vi "SR_FlipFlop_Example.vi"() -> ()   [LabVIEW 2019]
uses:
  <vilib>/Rock Robotics/WPI/ThirdParty/JAS_Junk/TrajLib/Trajectory_Library.lvlib
panel:
  in  "Set":bool
  in  "Reset":bool
  out "Output":bool
  out "NOT Output":bool
  out "Digital State Chart":cluster{dbl, dbl, dbl, dbl}(graph)
  # "S/R (Set/Reset) Flip-Flop Example"
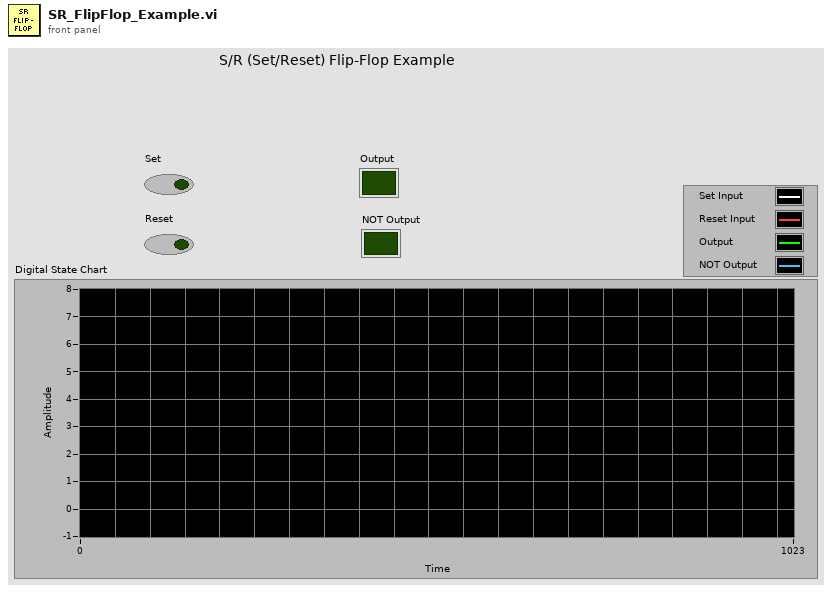
[diagram p1: front panel]
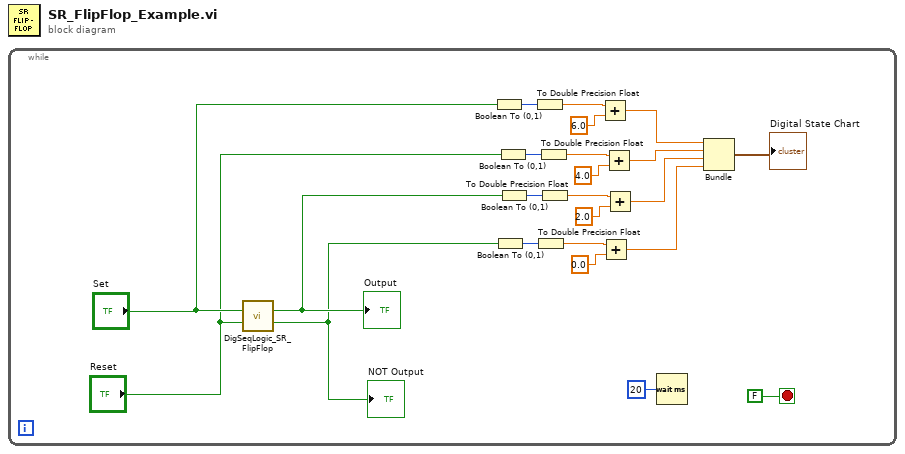
[diagram p0: block diagram]
diagram:
  n1 = while {
    stop <- FALSE stop-if-true
    n2 = call <vilib>:"DigSeqLogic_SR_FlipFlop.vi"("Set"="Set", "Reset"="Reset") -> ("Output"=w5:bool, "Inverse Output"=w4:bool)  [unwired: 12 in]
    "Output" <- w5
    "NOT Output" <- w4
    n3 = Boolean To (0,1)(Boolean="Set") -> (0, 1=w10:i16)
    n4 = Boolean To (0,1)(Boolean=w4) -> (0, 1=w11:i16)
    n5 = Boolean To (0,1)(Boolean="Reset") -> (0, 1=w13:i16)
    n6 = Boolean To (0,1)(Boolean=w5) -> (0, 1=w15:i16)
    n7 = To Double Precision Float(number=w10) -> (double precision float=w20:dbl)
    n8 = To Double Precision Float(number=w11) -> (double precision float=w12:dbl)
    n9 = To Double Precision Float(number=w13) -> (double precision float=w14:dbl)
    n10 = To Double Precision Float(number=w15) -> (double precision float=w16:dbl)
    n11 = Add(x=w20, y=6.0) -> (x+y=w21:dbl)
    n12 = Add(x=w12, y=0.0) -> (x+y=w19:dbl)
    n13 = Add(x=w14, y=4.0) -> (x+y=w17:dbl)
    n14 = Add(x=w16, y=2.0) -> (x+y=w18:dbl)
    n15 = Wait (ms)(milliseconds to wait=u32 20) -> ()  [unwired: 1 out]
    n16 = Bundle(w21, w17, w18, w19) -> (→"Digital State Chart":cluster{dbl, dbl, dbl, dbl})  [unwired: 1 in]
  }
